vi "Real Time Doppler Trigger.vi"() -> ()   [LabVIEW 2022 SP3]
doc: "Performs real-time Joint Time Frequency Analysis (JTFA) using Point By Point STFT. The signal is simulated by a sine wave plus Gaussian noise."
uses:
  <vilib>/DAQmx/read.llb/DAQmx Read (Analog 1D DBL 1Chan NSamp).vi
  <vilib>/measure/mamon.llb/Waveform Peak Detection for N Chan.vi
  <vilib>/DAQmx/miscellaneous.llb/DAQmx Fill In Error Info.vi
  <resource>/objmgr/daqmx.rc
  <vilib>/gmath/NI_Gmath.lvlib
  <vilib>/measure/NI_MAPro.lvlib
  <vilib>/ptbypt/NI_PtbyPt.lvlib
panel:
  out "Waveform Chart 2":dbl(graph)
  out "Boolean":bool
  out "Default Num samples 2":dbl=1024.0
  out "Waveform Chart":dbl[](graph)
  in  "Num samples to read":i32=128
  in  "window info":cluster{"type":u32, "window length":u32}={"type"=2, "window length"=128} {"window length" format="%0.0f"; "type" format="%0.0f"}
  in  "time-freq sampling":cluster{"time steps":i32, "freq bins":i32}={"time steps"=8, "freq bins"=64} {"freq bins" format="%0.0f"}
  out "DAQ error":errorcluster
  out "Default Num samples":dbl=1024.0
  in  "DAQmx Task Name":refnum<k21>="DopplerI"
  out "fs":dbl=24009.603841536613
  out "Moving STFT":dbl[][](graph)=[[0.001094360888039566, 0.00013614834701022508, 4.262180017532825e-05, 1.5585648701604173e-05, 3.134162842906104e-06, 2.326082981658581e-06, 2.1289896877143823e-06, 8.91914616333208e-07, 1.8886235442790794e-06, 1.8068601765114067e-06, 3.898964685694565e-07, 9.144281970757792e-07, 5.447387638180486e-07, 6.02068740943813e-07, 6.115001339763309e-07, 1.1965813401532138e-07, 1.5477007902705436e-07, 2.088202114351836e-07, 1.3411290490996363e-07, 4.1998924987119633e-07, 2.1463761155433114e-07, 3.984761280196815e-07, 3.3435082645157593e-07, 4.4556318865725325e-07, 1.2756947503811305e-08, 2.534322719751003e-07, 3.685415362664548e-07, 3.4912670193140304e-08, 6.098721724405258e-08, 5.126338264094161e-07, 8.317846709577462e-08, 2.01625476309565e-07], [0.001721398841689246, 0.00012002297797662927, 4.988517188375251e-05, 2.0758181860674842e-05, 6.7294368536517335e-06, 4.1665655806699735e-06, 3.10767358971238e-06, 7.927005340983228e-07, 1.8214022369235504e-06, 1.8487630086262888e-06, 4.2118199276998417e-07, 1.6272214070789419e-06, 9.989669293077178e-07, 9.903913973853158e-07, 8.457608612185379e-07, 1.459368539943136e-07, 1.242897175168758e-07, 1.9182720660584505e-07, 2.2616678558209973e-07, 8.389261517058944e-07, 3.8037508034286694e-07, 6.598276196337513e-07, 4.5221513383708193e-07, 5.4335822590479e-07, 2.405778406411523e-09, 2.720544179721034e-07, 5.273835018220648e-07, 5.612377324654226e-08, 1.2246611017238998e-07, 7.935894258329046e-07, 1.342609251455517e-07, 1.843069987360264e-07], [0.0025691417383821064, 0.00010634498820217139, 5.373888817297415e-05, 2.3283396548786586e-05, 2.5543913728760316e-06, 3.003974908617625e-06, 4.085394478082527e-06, 9.399061036739263e-07, 1.6247566668892612e-06, 2.076109203231579e-06, 5.874986218996305e-07, 1.1301727937716162e-06, 2.8043040255042393e-07, 7.77638671481409e-07, 9.231708246923019e-07, 1.663039759085766e-07, 8.736088808409817e-08, 1.9798838673960244e-07, 3.774280474012041e-07, 5.750228109234583e-07, 7.582076997391747e-08, 5.199222513619413e-07, 5.281219697635314e-07, 6.17960117272356e-07, 3.49040756449106e-08, 3.4623513174229915e-07, 7.745984185874923e-07, 4.261119537413692e-08, 1.2168243844369566e-08, 7.619350987953053e-07, 6.99778696042792e-08, 2.1714472570503207e-07], [0.0037196162264231747, 0.00011464702629985363, 3.478939999250269e-05, 1.1551409250127195e-05, 7.023261132550579e-06, 1.309018490190694e-06, 2.52625001291701e-06, 1.1251997728273287e-06, 1.3520605153636155e-06, 2.272553554934255e-06, 3.555126644500605e-07, 7.426425265125029e-07, 6.459105614298601e-07, 3.077812996406526e-07, 4.333274499308098e-07, 8.83525736805173e-08, 9.017800804759132e-08, 2.0884504699415092e-07, 2.687643436941776e-07, 8.100281928352659e-07, 2.2549119072791935e-07, 2.900591582361981e-07, 2.751239959573684e-07, 6.63328108309279e-07, 1.2484134023459545e-07, 4.045631568200311e-07, 5.904362956173025e-07, 1.6276360653125872e-08, 2.6621447636854646e-08, 3.9315018921089066e-07, 9.463333283349616e-09, 2.589630226525026e-07], [0.0052862183117654065, 0.0001500086228047357, 1.8743122542547287e-05, 1.7390698678170997e-05, 1.934115578576466e-06, 3.389862404932915e-06, 8.493856531160905e-07, 1.1565663307112253e-06, 1.0832554077386788e-06, 1.9964307853588788e-06, 7.060596369395313e-08, 1.0960255877625358e-06, 3.9739221244908476e-08, 6.68824277048617e-07, 7.80347180749919e-08, 3.0301731151953395e-09, 1.2643037638263145e-07, 1.761139114507215e-07, 6.329190962805437e-08, 1.0053733459929802e-06, 1.1612654031909524e-08, 4.933141054523801e-07, 6.665900014004507e-08, 5.612857282838687e-07, 2.480229882386457e-07, 3.964110011418273e-07, 3.5717749407424904e-07, 9.134128612409333e-10, 5.924331846513471e-08, 5.389548394336336e-07, 1.7042856461324752e-07, 2.942263695615956e-07], [0.007375566249462967, 0.00020781320741054365, 1.8896377158587012e-05, 1.2438083480672596e-05, 5.891060259937013e-06, 1.0249616280014546e-06, 1.495490003357021e-06, 8.933233102876175e-07, 9.642887512747178e-07, 1.2005030415895378e-06, 4.492507432816873e-09, 1.7807343296930487e-07, 2.4615076101858075e-07, 3.389638235550427e-07, 8.931083204013814e-08, 8.556030546448692e-08, 1.6136045214890274e-07, 1.2770075325260565e-07, 6.869866412646218e-08, 6.140445308410825e-07, 9.870791737425389e-08, 1.4656947954817808e-07, 1.0811448971139699e-07, 3.6015267070340454e-07, 3.673870693696251e-07, 3.0556667834264994e-07, 4.863359682539031e-07, 9.603263430924076e-08, 1.2724449192161079e-08, 2.8690371187297256e-07, 2.0361597563573386e-07, 2.6815839827019795e-07], [0.010037582300739437, 0.00028756425533620083, 1.3178241491357356e-05, 5.516706804342857e-06, 2.155689601815359e-06, 1.1308183073500112e-06, 1.6793829361274781e-06, 6.569360949589352e-07, 8.935178843369039e-07, 4.989326674147475e-07, 1.1398905409352133e-07, 2.650686421822063e-07, 7.75821989193354e-09, 1.695758157014865e-07, 1.3520329206898138e-07, 2.9389745985132634e-07, 1.935539823504375e-07, 9.24762560707347e-08, 1.1102338480736878e-07, 1.0701365721054256e-06, 1.520474631150245e-08, 3.1006289861498625e-07, 6.487238639519483e-08, 1.6848125449288758e-07, 4.350323772842084e-07, 1.9379051524071012e-07, 5.051369870864885e-07, 7.61967180213463e-08, 1.513164632526519e-07, 1.0046326477508161e-07, 2.860783404072479e-07, 2.136341147710858e-07], [0.01320752697674149, 0.0003906798791002739, 7.256816309359413e-06, 6.66503436417701e-06, 4.095796958398437e-06, 1.6385059099185539e-06, 9.912602790398427e-07, 5.052104068651639e-07, 7.62268340111471e-07, 2.1319677379256227e-07, 1.5557152079220307e-07, 7.558250851956254e-08, 5.7622193400427974e-08, 3.70427776715039e-07, 1.7370410009706696e-07, 5.01645059290002e-07, 1.7998093962451527e-07, 7.92189418077938e-08, 5.804168987884009e-08, 9.567623704405926e-07, 4.0224472117266505e-08, 3.121862871284105e-07, 1.3899877313260373e-08, 7.288105089665003e-08, 5.037709486298525e-07, 1.5740804100692967e-07, 3.7534588213385426e-07, 7.269272916429151e-08, 1.2381971739729912e-07, 9.499613589557532e-08, 5.388203410392133e-07, 2.1536118618037114e-07], [0.016641360655295916, 0.0005135921147339192, 9.672649092536564e-06, 3.528435491379866e-06, 2.515952554448743e-06, 1.059076150233268e-06, 7.019588163870297e-07, 4.7157280776282315e-07, 7.454954930454388e-07, 1.7056108780195567e-07, 1.3612179229209065e-07, 1.5476249558474082e-07, 6.936492371972343e-09, 2.581278094291483e-07, 1.2072832695021576e-07, 5.441663012736378e-07, 1.3136065438039482e-07, 5.569271761072047e-08, 1.2897033407888979e-08, 1.039408688415866e-06, 2.5650534025037807e-08, 4.069936872644806e-07, 7.584327688619238e-09, 3.989956677883438e-08, 5.073049750343691e-07, 1.8773463489072278e-07, 3.152596976687123e-07, 1.0447542645793628e-07, 2.2818004079645784e-07, 4.7798704439291756e-08, 6.240683946854536e-07, 2.628093377167218e-07], [0.019559538400380924, 0.0006522986444992266, 7.050209334806164e-06, 3.025954617511362e-06, 1.0558769704968564e-06, 6.339609886485917e-07, 5.595319458889885e-07, 6.283204189239914e-07, 5.546440702126862e-07, 8.296006985654146e-08, 2.630825023431389e-07, 4.1669061787528274e-07, 1.045894154092005e-08, 2.8429898245136214e-07, 1.8215060227797614e-07, 6.855484097303238e-07, 8.403106614382144e-08, 9.480595647488221e-08, 1.4831208455102909e-08, 9.472187143575412e-07, 5.360038497751101e-08, 4.505131760800129e-07, 4.8796507466537815e-08, 2.557609890192609e-08, 5.559640055649787e-07, 2.2848344718965918e-07, 2.5270117056734933e-07, 1.5045568601053217e-07, 3.7078322371304497e-07, 7.783550433821461e-08, 7.484364086980798e-07, 3.275132523404643e-07], [0.021494244570905808, 0.0007846727946098732, 6.184675816530151e-06, 1.7305869383009797e-06, 1.069219985298617e-06, 6.12710501354909e-07, 1.873846408025926e-07, 6.782856928586187e-07, 2.4790244411380344e-07, 2.2049111851566638e-08, 2.4718593672925535e-07, 8.247670587010853e-07, 2.263174629867135e-08, 1.2970551257407032e-07, 1.3604789096657862e-07, 8.833941785460749e-07, 7.262548260545466e-08, 1.2122538207565337e-07, 9.546980747770274e-09, 1.1648521191060645e-06, 6.728593912348535e-08, 6.918654745305801e-07, 8.356605918064671e-08, 3.8064280422133394e-08, 6.8048936852362e-07, 2.1691770171532672e-07, 1.705774944488577e-07, 1.410227894994945e-07, 3.512168520355811e-07, 1.2088200008764749e-07, 7.128680152094533e-07, 3.311452377082682e-07], [0.021834538601375617, 0.0009132708270981023, 4.762954640182631e-06, 2.904675144801502e-06, 2.3619782791028788e-07, 3.6958701836857e-07, 8.32419707815796e-08, 7.943593228809725e-07, 3.400219092552306e-08, 6.344923314146676e-08, 3.4262405568428036e-07, 1.0726653295668076e-06, 1.386178194086809e-07, 1.487629686560049e-07, 8.464574947307181e-08, 1.0480486999317514e-06, 1.0537729245219856e-07, 1.3080524258685719e-07, 7.957974667294046e-09, 9.84750207759903e-07, 2.223293164400145e-07, 6.51508273143423e-07, 1.1428367283025041e-07, 1.0771177674700865e-07, 8.377793442440358e-07, 1.8933145617385952e-07, 1.4647023770083747e-07, 1.4293515343336522e-07, 5.463989600302502e-07, 1.5789591699028659e-07, 5.388976047167701e-07, 2.744830072058196e-07], [0.02027075264322496, 0.0010176363000233004, 2.086817332575271e-06, 4.411296555099709e-06, 4.753821473708949e-07, 1.3622790284464284e-07, 4.6330939691700734e-08, 1.1453438489230337e-06, 2.3435481748755065e-08, 2.1282568998411246e-07, 4.1183340563617666e-07, 1.8202304397288517e-06, 2.1568571079514545e-07, 1.1517194390609561e-07, 9.180959596522808e-08, 1.1856194426485834e-06, 1.812707345831662e-07, 1.29361425359355e-07, 3.6496771588220228e-09, 9.541708362538903e-07, 3.1686343970949367e-07, 6.402547371875465e-07, 2.0601841016217165e-07, 2.1909285664173847e-07, 1.0081422702775782e-06, 1.4581738483108607e-07, 1.168373381425682e-07, 2.502798302669058e-07, 5.28785663599703e-07, 2.912725102389411e-07, 4.193892337538011e-07, 2.0150040140766965e-07], [0.017090492234061522, 0.0010732740079221026, 2.2254597398259896e-06, 5.404603538103045e-06, 1.661989870334601e-06, 3.535957897573737e-07, 1.2730553785345065e-07, 1.404256150414159e-06, 2.2115801967012277e-07, 3.703935638345307e-07, 2.2407219634483997e-07, 1.9121403602844935e-06, 5.001838166163123e-07, 5.825575375599882e-08, 1.644857808965838e-07, 1.1907932446435358e-06, 3.120330052441706e-07, 1.322215844867862e-07, 1.8611748818801512e-08, 9.017818859430856e-07, 6.408229846258784e-07, 6.411679693653395e-07, 3.029032624509245e-07, 3.3756214032392773e-07, 1.1479094837212408e-06, 1.189504822658614e-07, 4.566188980333111e-08, 2.4414154966742276e-07, 7.102612980452746e-07, 3.572156461622331e-07, 3.444664870756955e-07, 1.252382943892779e-07], [0.013020918886508522, 0.001053415093296641, 5.731983447061667e-06, 9.94770814486947e-06, 2.1592525039805973e-06, 4.17874386951995e-07, 3.9223657025803887e-07, 1.6614180052998163e-06, 5.37023897015944e-07, 4.745136559978608e-07, 4.647775894585193e-08, 1.959429604306375e-06, 5.345058369994718e-07, 1.1597148962683092e-07, 2.326095240458894e-07, 1.1568234199004301e-06, 4.340495717356648e-07, 1.2563380292947064e-07, 3.6047278968672736e-08, 6.55566773772697e-07, 7.025631648529937e-07, 4.095155091884898e-07, 3.0097023939681264e-07, 4.163744536335133e-07, 1.1518172084926495e-06, 9.570029152291775e-08, 2.2481912921916712e-08, 2.82145195933587e-07, 6.028780229838555e-07, 3.2048387217430433e-07, 1.9885563375499372e-07, 8.09511161045702e-08], [0.008874630864516245, 0.0009350147943119245, 7.2542226481728954e-06, 1.1397890874613508e-05, 4.199476902884821e-06, 1.3400312802795368e-06, 4.639684977584608e-07, 1.571135426515134e-06, 7.581565497218304e-07, 4.904883485888612e-07, 2.780369574180116e-08, 2.1512081860251544e-06, 8.403858951255982e-07, 1.829118375477539e-07, 2.0404884721082944e-07, 9.625332762332152e-07, 4.787893973481869e-07, 1.1518752509876138e-07, 2.7077096090588125e-08, 6.920831383998084e-07, 9.887499920664006e-07, 4.0011127839250414e-07, 2.0708581852845833e-07, 4.339838689687101e-07, 1.0250088536719626e-06, 9.094487998383664e-08, 4.459942481651092e-08, 3.7621491881412286e-07, 7.066116487401428e-07, 3.7951311828254433e-07, 7.624876527433804e-08, 5.461880032993973e-08], [0.0053697341232960116, 0.0007373961921656372, 6.906612675938378e-06, 9.07984383991257e-06, 2.8558807273323085e-06, 7.355089225505724e-07, 2.8818925432860377e-07, 1.3020845608710132e-06, 8.113736248485104e-07, 4.950042547458387e-07, 1.601134153240575e-08, 1.2045196861654555e-06, 5.239263158100703e-07, 7.217033926236346e-08, 1.5085489193997193e-07, 7.228062922204195e-07, 4.451338952196366e-07, 1.269667942160886e-07, 1.1823566334060046e-09, 4.10150541475801e-07, 6.558966476630186e-07, 2.2567247861043007e-07, 1.7463731759062225e-07, 3.9932992706828914e-07, 7.93550239124967e-07, 1.1051402031419618e-07, 2.2286957841935446e-08, 2.1998010052812614e-07, 4.218400431182435e-07, 2.3392474209765042e-07, 2.895897735653871e-08, 4.5720196411592524e-08]]
  in  "stop":bool
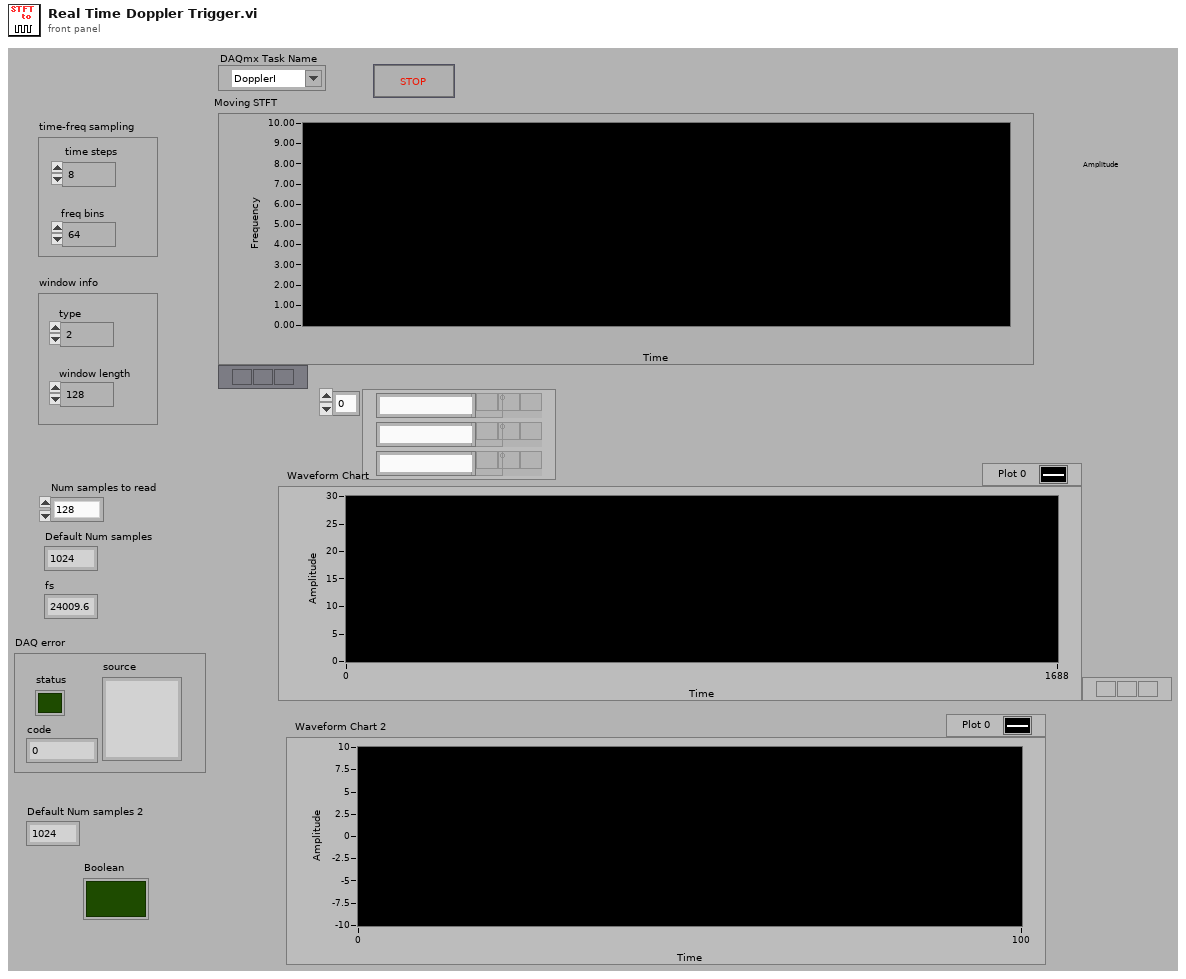
[diagram p1: front panel]
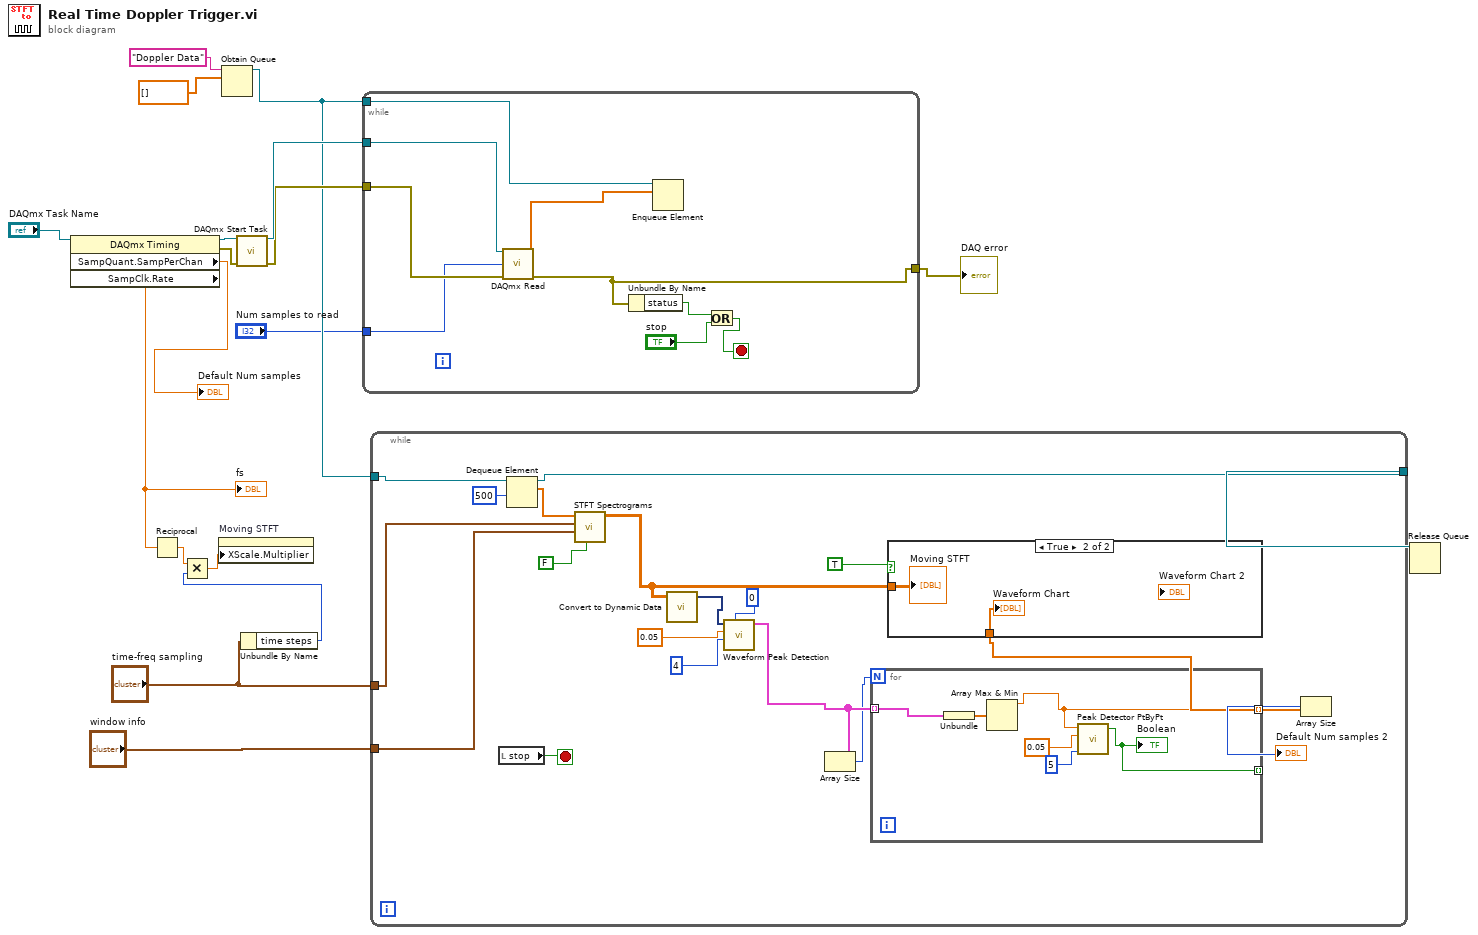
[diagram p0: block diagram]
diagram:
  n1 = property class="DAQmx Timing"(reference="DAQmx Task Name") -> (reference out=w17:refnum<k21>, error out=w16:errorcluster, "SampQuant.SampPerChan"=→"Default Num samples":dbl, "SampClk.Rate"=w12:dbl)  [unwired: 1 in]
  "fs" <- w12
  n2 = Reciprocal(x=w12) -> (1/x=w3:dbl)
  n3 = Obtain Queue(name (unnamed)="Doppler Data", element data type=dbl[] [] ("Y")) -> (queue out=w10:refnum<queue>)  [unwired: 3 in, 2 out]
  n4 = call <vilib>:"DAQmx Start Task.vi"("task/channels in"=w17, "error in"=w16) -> ("task out"=w15:refnum<k21>, "error out"=w14:errorcluster)  [unwired: 12 out]
  n5 = Unbundle By Name("time-freq sampling") -> ("time steps"=w2:i32)
  n6 = Multiply(x=w3, y=w2) -> (x*y=w1:dbl)
  n7 = property on="Moving STFT" class="IntChart (strict)"("XScale.Multiplier"=w1) -> ()  [unwired: 2 in, 2 out]
  n8 = while {
    tunnel: w15 -> [w27]
    tunnel: [w21] -> w18
    tunnel: w14 -> [w26]
    tunnel: w10 -> [w25]
    tunnel: "Num samples to read" -> [w24]
    stop <- w22 stop-if-true
    n9 = call-poly <vilib>:"DAQmx Read.vi"("task/channels in"=w27, "number of samples per channel"=w24, "error in"=w26) -> ("data"=w19:dbl[], "error out"=w21:errorcluster)  [unwired: 11 out]
    n10 = Unbundle By Name(w21) -> ("status"=w20:bool)
    n11 = Enqueue Element(queue=w25, element=w19) -> ()  [unwired: 1 in, 4 out]
    n12 = Or(x=w20, y="stop") -> (x .or. y?=w22:bool)
  }
  "DAQ error" <- w18
  n13 = while {
    tunnel: w10 -> [w40]
    tunnel: "time-freq sampling" -> [w45]
    tunnel: "window info" -> [w44]
    tunnel: [w39] -> w7
    stop <- w29 stop-if-true
    n14 = local read "stop"() -> (w29:bool)
    n15 = Dequeue Element(queue=w40, timeout in ms (-1)=500) -> (queue out=w39:refnum<queue>, element=w42:dbl[])  [unwired: 1 in, 2 out]
    n16 = call <vilib>:"STFT Spectrograms.vi"("energy conservation?"=FALSE, "window info"=w44, "time-freq sampling info"=w45, "X"=w42) -> ("STFT Spectrogram {X}"=w37:dbl[][])  [unwired: 2 in, 5 out]
    n17 = call "Convert to Dynamic Data"("2D Array"=w37) -> ("Dynamic Data Type"=w31:dynamicdata)  [unwired: 3 out]
    n18 = call-poly <vilib>:"Waveform Peak Detection.vi"("peaks/valleys"=u32 0 ("milliseconds to wait"), "width"=u32 4 ("milliseconds to wait"), "threshold"=0.05 ("Y Scale.Range:Minimum"), "Signals In"=w31) -> ("Locations"=w35:cluster{"Locations":dbl[]}[])  [unwired: 3 in, 4 out]
    n19 = Array Size(array=w35) -> (size(s)=w33:i32)
    n20 = for {
      N: w33 -> [_]
      tunnel: [w46] -> w28 mode=indexing
      tunnel: w35 -> [w50] mode=indexing
      tunnel: [w47] -> _ mode=indexing
      n21 = Unbundle(w50) -> ("Locations"=w51:dbl[])
      n22 = Array Max & Min(array=w51) -> (max value=w46:dbl)  [unwired: 3 out]
      n23 = call <vilib>:"Peak Detector PtByPt.vi"("x"=w46, "threshold peak"=0.05 ("Y Scale.Range:Minimum"), "width"=u32 5 ("milliseconds to wait")) -> ("peak"=w47:bool)  [unwired: 2 in, 2 out]
      "Boolean" <- w47
    }
    n24 = case shown="True" TRUE {
      tunnel: w37 -> [_ w53]
      tunnel: w28 -> [_ w52]
      frame False {
      }
      frame True {
        "Moving STFT" <- w53
        "Waveform Chart" <- w52
      }
    }
    n25 = Array Size(array=w28) -> (size(s)=→"Default Num samples 2":i32)
  }
  n26 = Release Queue(queue=w7) -> ()  [unwired: 1 in, 4 out]
